vi "refAssemblies.vi"(8 "error in (no error)":errorcluster, 11 "Document in":refnum<class "Document.lvclass">) -> (0 "error out":errorcluster, 3 "Document out":refnum<class "Document.lvclass">)   [LabVIEW 2017, in "LabVIEW NPOI.lvlib" / "Document.lvclass"]
doc: "This VI does nothing, it is used to make sure that all NPOI Assemblies are included during build process."
uses:
  Document.lvclass
  ICSharpCode.SharpZipLib
  C:/Users/Neo/Desktop/Dev_Tools_BR/LabVIEW_NPOI/src/lib/NPOI 2.1.1/NPOI.dll
  lib/NPOI 2.1.1/NPOI.dll
  C:/Users/Neo/Desktop/Dev_Tools_BR/LabVIEW_NPOI/src/lib/NPOI 2.1.1/NPOI.OOXML.dll
  lib/NPOI 2.1.1/NPOI.OOXML.dll
  C:/Users/Neo/Desktop/Dev_Tools_BR/LabVIEW_NPOI/src/lib/NPOI 2.1.1/NPOI.OpenXml4Net.dll
  lib/NPOI 2.1.1/NPOI.OpenXml4Net.dll
  C:/Users/Neo/Desktop/Dev_Tools_BR/LabVIEW_NPOI/src/lib/NPOI 2.1.1/NPOI.OpenXmlFormats.dll
  lib/NPOI 2.1.1/NPOI.OpenXmlFormats.dll
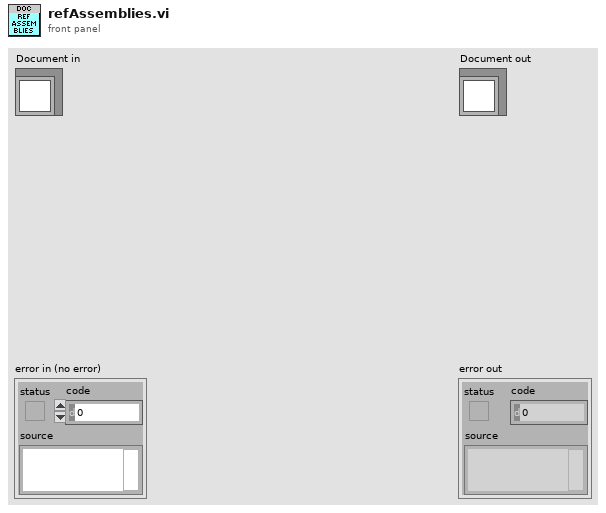
[diagram p1: front panel]
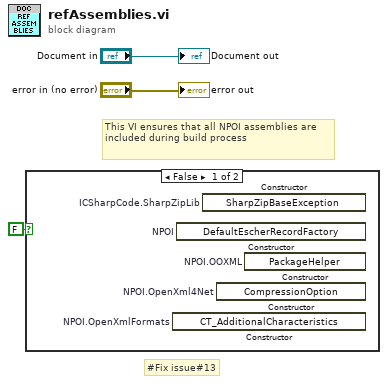
[diagram p0: block diagram]
diagram:
  # "This VI ensures that all NPOI assemblies are included during build process"
  # "#Fix issue#13"
  n1 = case shown="False" FALSE {
    frame False {
      n2 = constructor on="NPOI.OpenXmlFormats" class="CT_AdditionalCharacteristics"() -> ()  [unwired: 3 in, 3 out]
      n3 = constructor on="NPOI" class="DefaultEscherRecordFactory"() -> ()  [unwired: 3 in, 3 out]
      n4 = constructor on="ICSharpCode.SharpZipLib" class="SharpZipBaseException"() -> ()  [unwired: 3 in, 3 out]
      n5 = constructor on="NPOI.OpenXml4Net" class="CompressionOption"() -> ()  [unwired: 3 in, 3 out]
      n6 = constructor on="NPOI.OOXML" class="PackageHelper"() -> ()  [unwired: 3 in, 3 out]
    }
    frame True {
    }
  }
  "error out" <- "error in (no error)"
  "Document out" <- "Document in"
